vi "GetIpmStatus.vi"(4 "error in (no error)":errorcluster, 7 "axis in":cluster{"keyHandle":u32, "nodeId":u16}={"keyHandle"=0, "nodeId"=1}) -> (0 "error out":errorcluster, 2 "IPM status":T1, 3 "axis out":cluster{"keyHandle":u32, "nodeId":u16}={"keyHandle"=0, "nodeId"=1})   [LabVIEW 2019, in "maxonEPOS.lvlib"]
doc: "The function <B>VCS_GetIpmStatus</B> returns all IPM warning and error states."
uses:
  Examples/maxonEPOS.lvlib
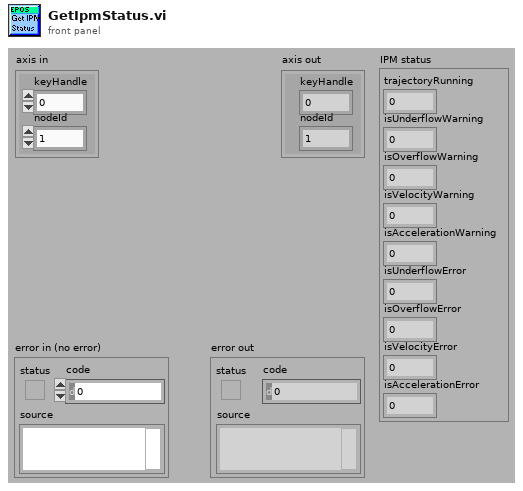
[diagram p1: front panel]
types:
  T1 = cluster{"trajectoryRunning":i32, "isUnderflowWarning":i32, "isOverflowWarning":i32, "isVelocityWarning":i32, "isAccelerationWarning":i32, "isUnderflowError":i32, "isOverflowError":i32, "isVelocityError":i32, "isAccelerationError":i32}
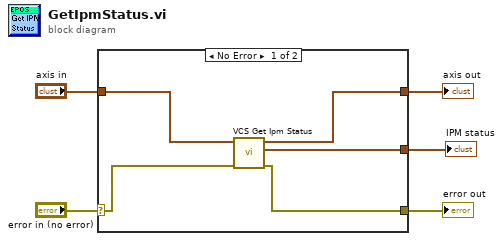
[diagram p0: block diagram]
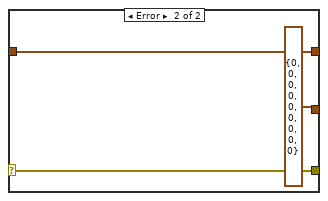
[diagram p2: hidden frame]
diagram:
  n1 = case shown="No Error" "error in (no error)" {
    selector: "error in (no error)" -> [w10 w13]
    tunnel: [w6 w13] -> w4
    tunnel: [w8 w12] -> w3
    tunnel: "axis in" -> [w9 w12]
    tunnel: [w7 T1 {"trajectoryRunning"=0, "isUnderflowWarning"=0, "isOverflowWarning"=0, "isVelocityWarning"=0, "isAccelerationWarning"=0, "isUnderflowError"=0, "isOverflowError"=0, "isVelocityError"=0, "isAccelerationError"=0} ("IPM status")] -> w1
    frame No Error {
      n2 = call "VCS Get Ipm Status.vi"("error in (no error)"=w10, "axis in"=w9) -> ("error out"=w6:errorcluster, "IPM status"=w7:T1, "axis out"=w8:cluster{"keyHandle":u32, "nodeId":u16})  [unwired: 5 in]
    }
    frame Error {
    }
  }
  "error out" <- w4
  "axis out" <- w3
  "IPM status" <- w1
